vi "CCSA RPJ SLJC PF SubVI004.vi"(1 "Dato":string="Refresco: ", 3 "Nombre imagen":string="s", 5 "Class":string, 7 "Dato 2":string, 9 "Distance (Pixels)":dbl, 11 "Dato 3":string, 12 "Refnum in":T1, 13 "empty?":bool, 14 "number":i32) -> (4 "new picture":picture)   [LabVIEW 2021]
doc: "Coloca datos en la imagen y luego la guarda"
uses:
  <vilib>/vision/Image Controls.llb/IMAQ Image.ctl
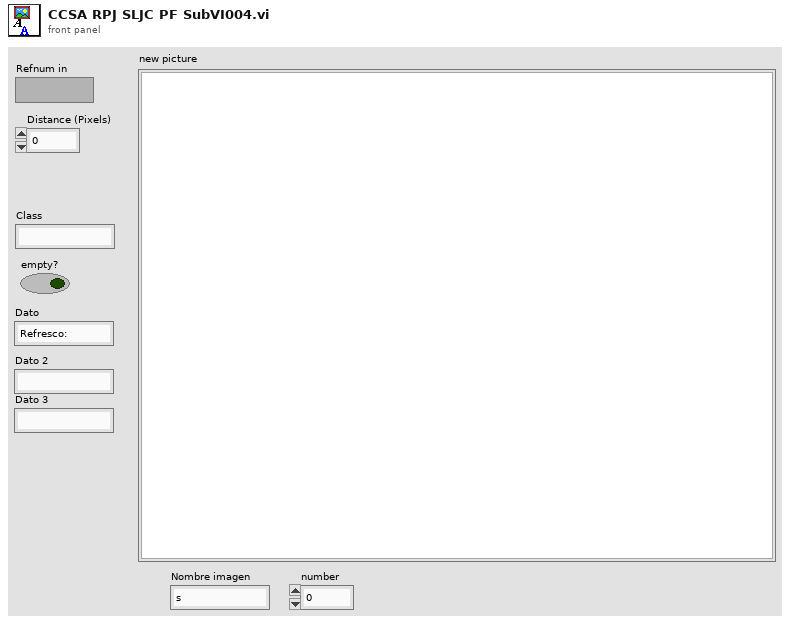
[diagram p1: front panel]
types:
  T1 = typedef "IMAQ Image.ctl" = refnum<image>
  T2 = enum16{"User-specified Font", "Application Font", "System Font", "Dialog Font"}
  T3 = cluster{"Font Name:":string, "Size":i16, "Strikeout?":bool, "Italic?":bool, "Underline?":bool, "Outline?":bool, "Shadow?":bool, "Bold?":bool}
  T4 = cluster{"left":i16, "top":i16, "right":i16, "bottom":i16}
  T5 = typedef "imagedata.ctl" = cluster{"image type":i32, "image depth":i32, "image":u8[], "mask":u8[], "colors":u32[], "Rectangle":cluster{"left":i16, "top":i16, "right":i16, "bottom":i16}}
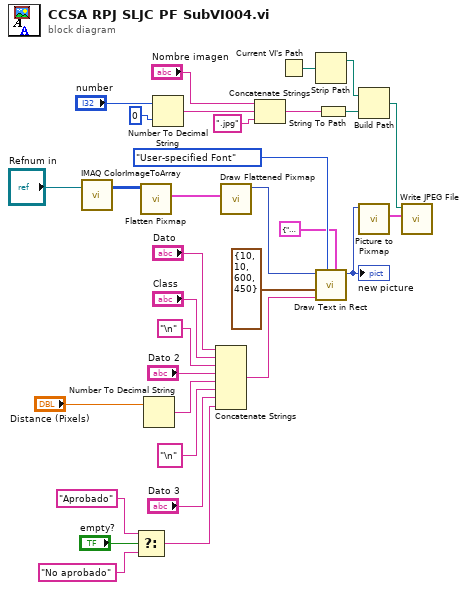
[diagram p0: block diagram]
diagram:
  n1 = call "IMAQ ColorImageToArray"("Image"="Refnum in") -> ("Image Pixels (U32)"=w19:u32[][])  [unwired: 3 in, 2 out]
  n2 = Select(t="Aprobado", s="empty?", f="No aprobado") -> (s? t:f=w5:string)
  n3 = call <vilib>:"Flatten Pixmap.vi"("24-bit pixmap"=w19) -> ("image data"=w20:T5)  [unwired: 10 in]
  n4 = Number To Decimal String(number="Distance (Pixels)") -> (decimal integer string=w3:string)  [unwired: 1 in]
  n5 = Number To Decimal String(number="number", width (-)=i16 0) -> (decimal integer string=w13:string)
  n6 = Concatenate Strings("Dato", "Class", "\n" ("string"), "Dato 2", w3, "\n" ("string"), "Dato 3", w5) -> (w31:string)
  n7 = call <vilib>:"Draw Flattened Pixmap.vi"("image data"=w20) -> ("new picture"=w21:picture)  [unwired: 8 in]
  n8 = Concatenate Strings("Nombre imagen", w13, ".jpg" ("string")) -> (w14:string)
  n9 = Current VI's Path() -> (path=w12:path)
  n10 = Strip Path(path=w12) -> (stripped path=w11:path)  [unwired: 1 out]
  n11 = call <vilib>:"Draw Text in Rect.vi"("[user-specified font]"=T3 {"Font Name:"="Arial", "Size"=20, "Strikeout?"=FALSE, "Italic?"=TRUE, "Underline?"=FALSE, "Outline?"=FALSE, "Shadow?"=TRUE, "Bold?"=TRUE}, "desired font(Application)"=T2."User-specified Font", "text"=w31, "rect"=T4 {"left"=10, "top"=10, "right"=600, "bottom"=450}, "picture"=w21) -> ("new picture"=w17:picture)  [unwired: 6 in]
  "new picture" <- w17
  n12 = String To Path(string=w14) -> (path=w15:path)
  n13 = Build Path(base path=w11, name or relative path=w15) -> (appended path=w7:path)
  n14 = call <vilib>:"Picture to Pixmap.vi"("picture"=w17) -> ("image data"=w16:T5)  [unwired: 9 in, 1 out]
  n15 = call <vilib>:"Write JPEG File.vi"("image data"=w16, "path to JPEG file"=w7) -> ()  [unwired: 8 in, 2 out]
